vi "pubEvent.vi"(8 "error in (no error)":errorcluster, 9 "variant":variant, 10 "name":string, 11 "SalProcess in":refnum<class "SalProcess.lvclass">) -> (0 "error out":errorcluster, 2 "function return":i32, 3 "SalProcess out":refnum<class "SalProcess.lvclass">)   [LabVIEW 2018, in "SalProcess.lvclass"]
doc: "Publish the event."
uses:
  SalProcess.lvclass
  SalProcess.lvclass/SalProcess.ctl
  LibReader/LibReader.lvclass
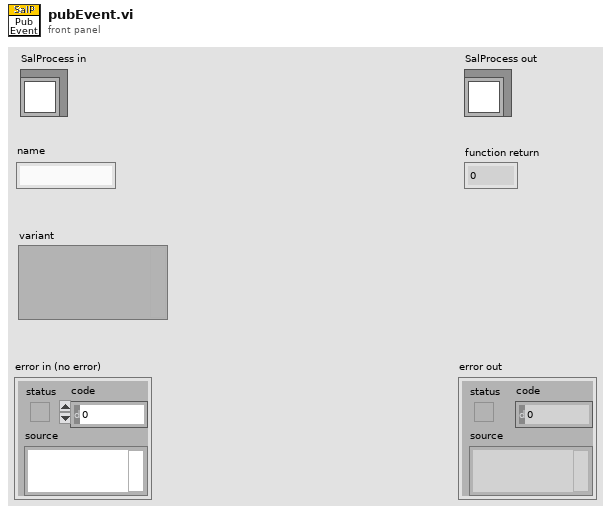
[diagram p1: front panel]
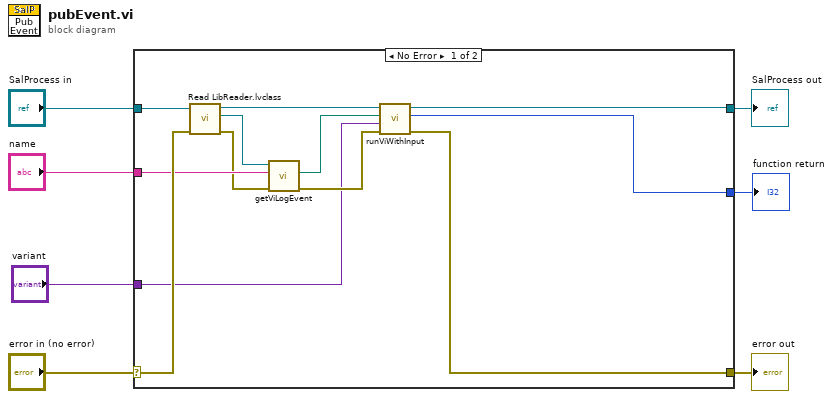
[diagram p0: block diagram]
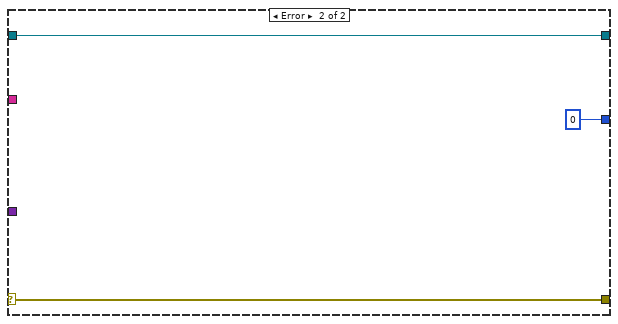
[diagram p2: hidden frame]
diagram:
  n1 = case shown="No Error" "error in (no error)" {
    selector: "error in (no error)" -> [w18 w22]
    tunnel: [w10 w22] -> w6
    tunnel: [w9 w21] -> w4
    tunnel: "SalProcess in" -> [w19 w21]
    tunnel: "name" -> [w16 _]
    tunnel: "variant" -> [w12 _]
    tunnel: [w8 0 ("function return")] -> w1
    frame No Error {
      n2 = call "Read LibReader.lvclass.vi"("error in (no error)"=w18, "SalProcess in"=w19) -> ("error out"=w15:errorcluster, "LibReader.lvclass"=w17:refnum<class "LibReader.lvclass">, "SalProcess out"=w14:refnum<class "SalProcess.lvclass">)  [unwired: 7 in]
      n3 = call "getViLogEvent.vi"("error in (no error)"=w15, "name"=w16, "LibReader in"=w17) -> ("error out"=w13:errorcluster, "pathViLogEvent"=w11:path)  [unwired: 6 in, 1 out]
      n4 = call "runViWithInput.vi"("error in (no error)"=w13, "variant"=w12, "vi path"=w11, "SalProcess in"=w14) -> ("error out"=w10:errorcluster, "function return"=w8:i32, "SalProcess out"=w9:refnum<class "SalProcess.lvclass">)  [unwired: 5 in]
    }
    frame Error {
    }
  }
  "error out" <- w6
  "SalProcess out" <- w4
  "function return" <- w1
